vi "更新关键字.vi"(8 "错误输入":errorcluster caption="错误输入（无错误）", 9 "变量函数":string[](array[string]), 10 "引用 2":refnum<k24>, 11 "引用":refnum<k24>) -> (0 "错误输出":errorcluster, 2 "引用输出 2":refnum<k24>, 3 "引用输出":refnum<k24>)   [LabVIEW 2018]
uses:
  ScintillaNET.dll
  AutocompleteMenu-ScintillaNET.dll
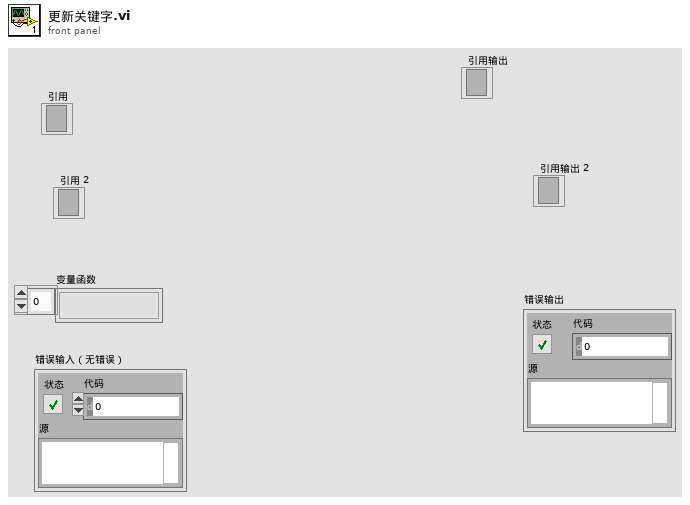
[diagram p1: front panel]
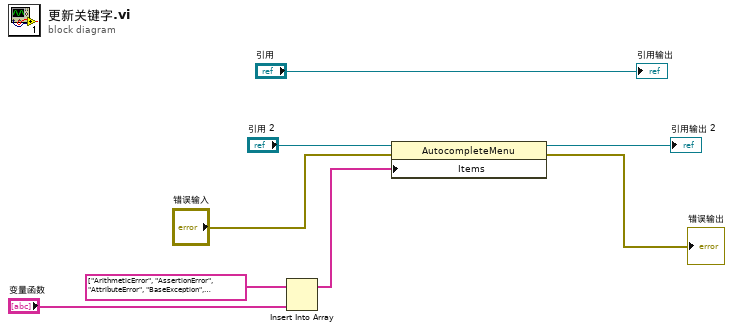
[diagram p0: block diagram]
diagram:
  n1 = Insert Into Array(array=string[] ["ArithmeticError", "AssertionError", "AttributeError", "BaseException", "BufferError", "BytesWarning", "DeprecationWarning", "EOFError", "EnvironmentError", "Exception", "False", "FloatingPointError", "FutureWarning", "GeneratorExit", "IOError", "ImportError", "ImportWarning", "IndentationError", "IndexError", "KeyError", "KeyboardInterrupt", "LookupError", "MemoryError", "NameError", "None", "NotImplementedError", "OSError", "OverflowError", "PendingDeprecationWarning", "ReferenceError", "RuntimeError", "RuntimeWarning", "StandardError", "StopIteration", "SyntaxError", "SyntaxWarning", "SystemError", "SystemExit", "TabError", "True", "TypeError", "UnboundLocalError", "UnicodeDecodeError", "UnicodeEncodeError", "UnicodeError", "UnicodeTranslateError", "UnicodeWarning", "UserWarning", "ValueError", "Warning", "ZeroDivisionError", "abs", "add", "all", "and", "any", "append", "apply", "as", "as_integer_ratio", "assert", "basestring", "bin", "bit_length", "bool", "break", "buffer", "bytearray", "bytes", "callable", "capitalize", "center", "chr", "class", "classmethod", "clear", "close", "cmp", "coerce", "compile", "complex", "conjugate", "continue", "copy", "count", "decode", "def", "del", "delattr", "deleter", "dict", "difference", "difference_update", "dir", "discard", "divmod", "elif", "else", "encode", "endswith", "enumerate", "eval", "except", "exec", "execfile", "expandtabs", "extend", "file", "fileno", "filter", "finally", "find", "float", "flush", "for", "format", "from", "fromhex", "fromkeys", "frozenset", "get", "getattr", "getter", "global", "globals", "has_key", "hasattr", "hash", "hex", "id", "if", "import", "in", "index", "indices", "input", "insert", "int", "intern", "intersection", "intersection_update", "is", "is_integer", "isalnum", "isalpha", "isatty", "isdecimal", "isdigit", "isdisjoint", "isinstance", "islower", "isnumeric", "isspace", "issubclass", "issubset", "issuperset", "istitle", "isupper", "items", "iter", "iteritems", "iterkeys", "itervalues", "join", "keys", "lambda", "len", "list", "ljust", "locals", "long", "lower", "lstrip", "map", "max", "memoryview", "min", "mro", "next", "not", "object", "oct", "open", "or", "ord", "partition", "pass", "pop", "popitem", "pow", "print", "property", "raise", "range", "raw_input", "read", "readinto", "readline", "readlines", "reduce", "reload", "remove", "replace", "repr", "return", "reverse", "reversed", "rfind", "rindex", "rjust", "round", "rpartition", "rsplit", "rstrip", "seek", "set", "setattr", "setdefault", "setter", "slice", "sort", "sorted", "split", "splitlines", "startswith", "staticmethod", "str", "strip", "sum", "super", "swapcase", "symmetric_difference", "symmetric_difference_update", "tell", "title", "tobytes", "tolist", "translate", "truncate", "try", "tuple", "type", "unichr", "unicode", "union", "update", "upper", "values", "vars", "viewitems", "viewkeys", "viewvalues", "while", "with", "write", "writelines", "xrange", "xreadlines", "yield", "zfill", "zip"] ("数组"), new element="变量函数") -> (w4:string[])  [unwired: 1 in]
  n2 = property class="AutocompleteMenu"(reference="引用 2", error in="错误输入", "Items"=w4) -> (reference out=→"引用输出 2":refnum<k24>, error out=→"错误输出":errorcluster)
  "引用输出" <- "引用"
